vi "EventLoop.Mathematica.vi"(0 "Ctrls":refnum<vi>[](array[refnum]), 1 "Name":string, 2 "Path":path) -> ()   [LabVIEW 2014]
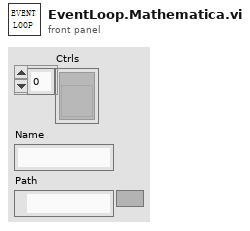
[diagram p1: front panel]
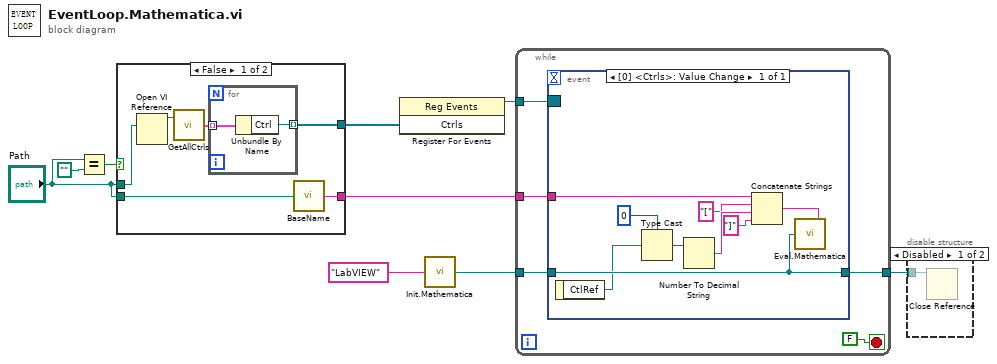
[diagram p0: block diagram]
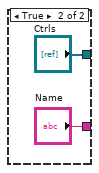
[diagram p2: hidden frame]
diagram:
  n1 = Equal?(x="Path", y=path "") -> (x = y?=w7:bool)
  n2 = case shown="False" w7 {
    tunnel: [w12 "Ctrls"] -> w6
    tunnel: [w11 "Name"] -> w3
    tunnel: "Path" -> [w13 _]
    tunnel: "Path" -> [w10 _]
    frame False {
      n3 = Open VI Reference(vi path=w13) -> (vi reference=w14:refnum<vi>)  [unwired: 5 in, 1 out]
      n4 = call "GetAllCtrls.vi"("VI"=w14) -> ("Ctrls"=w15:cluster{"Name":string, "Ctrl":refnum<vi>}[])  [unwired: 1 in]
      n5 = for {
        tunnel: w15 -> [w17] mode=indexing
        tunnel: [w16] -> w12 mode=indexing
        n6 = Unbundle By Name(w17) -> ("Ctrl"=w16:refnum<vi>)
      }
      n7 = call "BaseName.vi"("Path"=w10) -> ("Name"=w11:string)
    }
    frame True {
    }
  }
  n8 = register-events(w6) -> (reference out=w9:refnum<event-registration>)  [unwired: 2 in, 1 out]
  n9 = call "Init.Mathematica.vi"("Name"="LabVIEW" ("LinkName")) -> ("reference"=w2:refnum<k24>)
  n10 = while {
    tunnel: w2 -> [w23]
    tunnel: w9 -> [w22]
    tunnel: [w21] -> w4
    tunnel: w3 -> [w20]
    stop <- FALSE stop-if-true
    n11 = event shown="[0] <Ctrls>: Value Change" {
      selector: w22 -> [_]
      dyn-events: _ -> [_]
      timeout: _ -> [_]
      tunnel: w23 -> [w33]
      tunnel: [w33] -> w21
      tunnel: w20 -> [w25]
      event Value Change {
        n12 = event-data() -> ("CtlRef"=w31:refnum<vi>)  [unwired: 1 in]
        n13 = Type Cast(type=u32 0, x=w31) -> (*(type *) &x=w30:u32)
        n14 = Number To Decimal String(number=w30) -> (decimal integer string=w29:string)  [unwired: 1 in]
        n15 = Concatenate Strings(w25, "[" ("string"), w29, "]" ("string")) -> (w26:string)
        n16 = call "Eval.Mathematica.vi"("input"=w26, "reference"=w33) -> ()
      }
    }
  }
  n17 = disable-structure shown="Disabled" {
    disable-tunnel: w4 -> [w34 _]
    frame Disabled {
      n18 = Close Reference(reference=w34) -> ()  [unwired: 1 in, 1 out]
    }
    frame Enabled {
    }
  }
